vi "variantCtrlStepFunction.vi"(4 "isRequired (T)":bool=TRUE, 6 "menu in (get)":enum16{"get", "set"}(ring), 8 "error in":errorcluster, 9 "StepFunction":T1, 11 "variant in":variant) -> (0 "error out":errorcluster, 1 "StepFunction":T1, 2 "found/replaced":bool, 3 "variant out":variant)   [LabVIEW 2024]
uses:
  controls/type.StepFunction.ctl
  controls/typeStepVarients.ctl
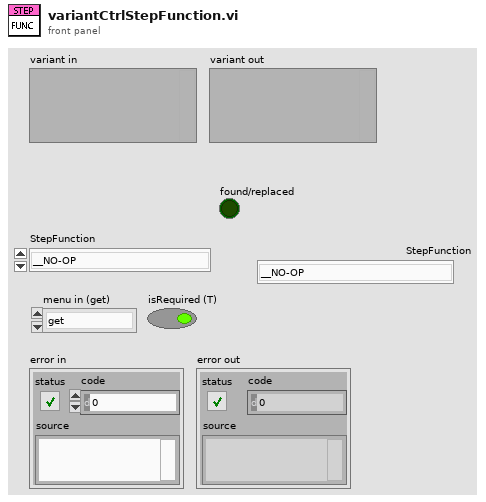
[diagram p1: front panel]
types:
  T1 = typedef "type.StepFunction.ctl" = enum16{"__NO-OP", "_DELAY_LOAD", "_DELAY_COMPARE", "_JUMP", "_COMPLETE", "_COMPARE", "_LOG_MESSAGE", "_LOG_LAST_REPORT", "_SCHEDULE", "_SCHED_DAILY", "CLK_COMPARE", "PROC_START", "PROC_STOP", "PROC_LOAD", "PROC_COMPLETION_CHECK", "PROC_COMPLETION_LOAD", "_IO_READ", "_IO_READ_MANY", "_IO_WRITE", "_IO_WRITE_BY_REG", "_IO_GET_OUTPUT", "_OCS_CHECK", "_OCS_RECORD", "_GET_RH", "_GET_ACC_UV", "_GET_WD", "_GET_WS", "_REC_DELETE", "_REC_MOVE", "_REC_COPY", "_IRR_CHECK", "UNIT_CHECK", "UNIT_SAMPLE", "UNIT_DOSE"}
  T2 = typedef "typeStepVarients.ctl" = enum16{"stepNameID", "stepFunction", "stepReport", "stepSetpoint", "stepPointer", "stepProcPointer", "stepIoPointer", "stepIoValue", "stepFilePointer", "stepMessage", "stepTimeString", "stepNumReg", "stepStrReg", "stepSeconds", "stepUnitDoseParams", "stepUnitIndex"}
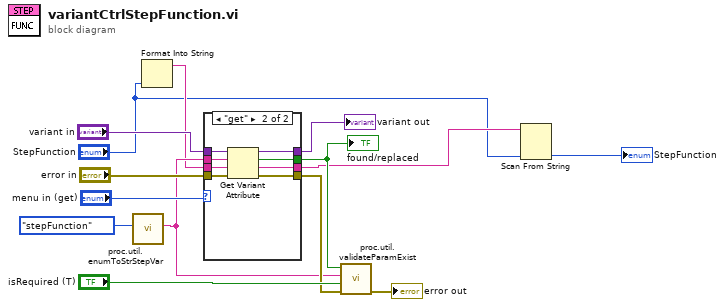
[diagram p0: block diagram]
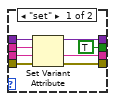
[diagram p2: hidden frame]
diagram:
  n1 = call "proc.util.enumToStrStepVar.vi"("Step var"=typeStepVarients."stepFunction" ("proc var")) -> ("String"=w5:string)  [unwired: 10 in]
  n2 = Format Into String("StepFunction") -> (resulting string=w4:string)  [unwired: 3 in, 1 out]
  n3 = case shown="\"get\"" "menu in (get)" {
    tunnel: "error in" -> [w21 w29]
    tunnel: w4 -> [w16 w28]
    tunnel: "variant in" -> [w20 w27]
    tunnel: [w19 w26] -> w8
    tunnel: [TRUE w25] -> w9
    tunnel: [w18 w24] -> w12
    tunnel: w5 -> [w17 w23]
    tunnel: [w16 w22] -> w3
    frame "set" {
      n4 = Set Variant Attribute(Variant=w20, name=w17, value=w16, error in=w21) -> (Variant out=w18:variant, error out=w19:errorcluster)  [unwired: 1 out]
    }
    frame "get" {
      n5 = Get Variant Attribute(Variant=w27, name=w23, default value (empty Variant)=w28, error in=w29) -> (duplicate Variant=w24:variant, found=w25:bool, value=w22:string, error out=w26:errorcluster)
    }
  }
  "found/replaced" <- w9
  "variant out" <- w12
  n6 = call "proc.util.validateParamExist.vi"("error in"=w8, "isRequired"="isRequired (T)", "Param Label"=w5, "isFound"=w9) -> ("error out"=→"error out":errorcluster)  [unwired: 7 in]
  n7 = Scan From String(input string=w3, default 1="StepFunction") -> (output 1=→"StepFunction":T1)  [unwired: 3 in, 3 out]
